vi "Main_TopLevel_1.vi"() -> ()   [LabVIEW 2010]
doc: "Use this template to create an application that executes until you click the Stop button. Unlike the Single Loop Application VI that uses polling, this VI uses the Event Structure."
uses:
  Main_cluster.ctl
  PI E710 Stage.lvlib
panel:
  in  "Center cursor":bool
  in  "Skip scan":bool
  out "Timetrace":dbl[](graph)
  in  "Tab Control":enum32{"Main", "Stage", "Spectrometer"}(tab)
  in  "File":path
  in  "Timetrace length (s)":i32=1024
  in  "Counter Device":tag="APD_Count"
  in  "Acquisition time (s)":dbl=1.0
  in  "Save as":enum16{"", "ASCII", "OriginLab", "Matlab"}(ring)
  in  "Map Geometry":T1
  out "Stage Identification string":string
  out "Position [micrometers]":dbl[](array[numeric]) format="%.6f"
  in  "Scan as cursor":bool
  in  "Position list":dbl[][](array[numeric])
  in  "Stop scan":bool
  in  "Clear list":bool
  in  "Scan":bool
  in  "Move to cursor":bool
  in  "Add to list":bool
  in  "Measure timetraces":bool
  in  "quit":bool
  out "Intensity Graph":dbl[][](graph)
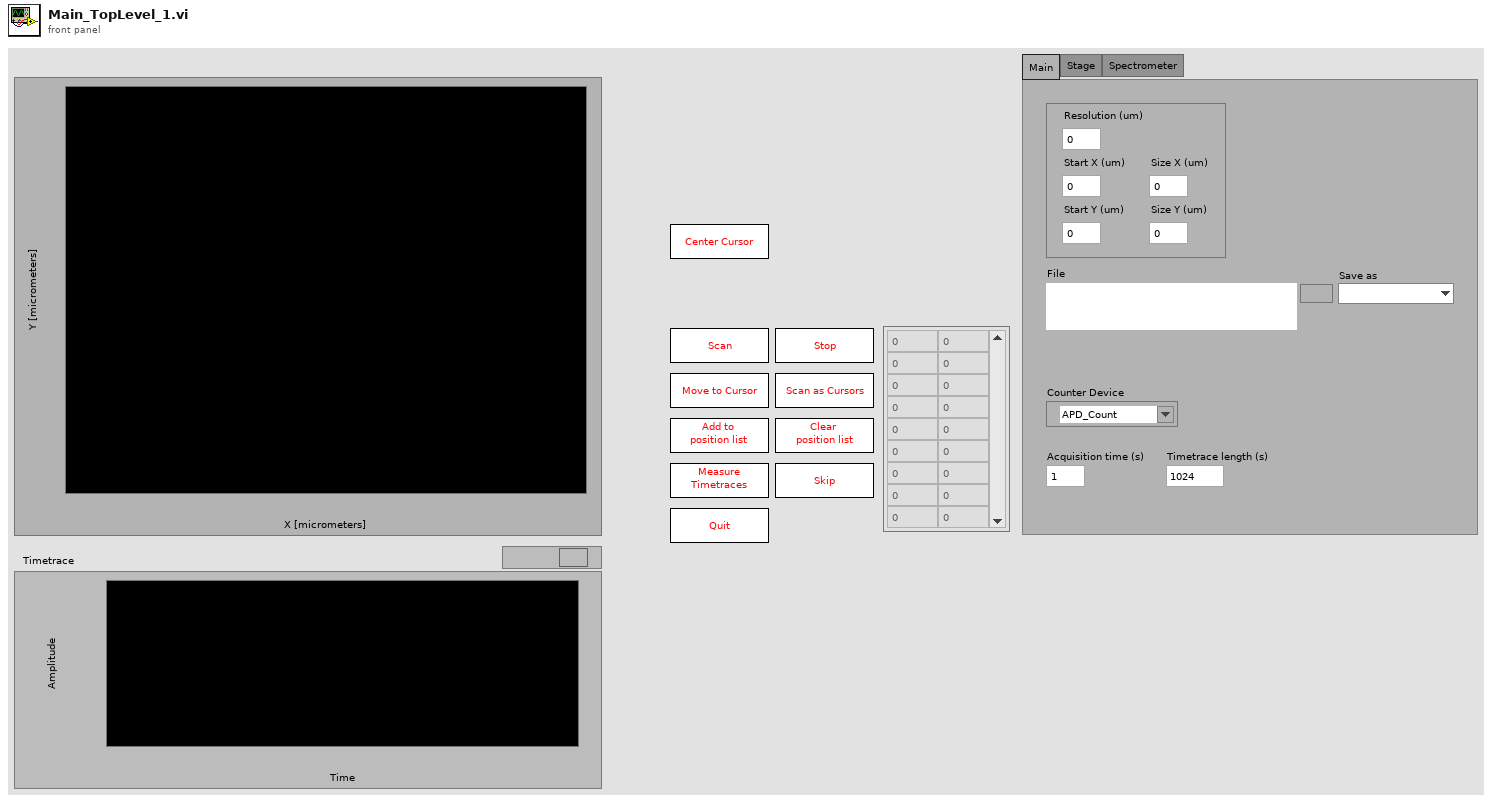
[diagram p1: front panel]
types:
  T1 = cluster{"Size Y (um)":dbl, "Size X (um)":dbl, "Start Y (um)":dbl, "Start X (um)":dbl, "Resolution (um)":dbl}
  T2 = typedef "Main_cluster.ctl" = cluster{"Task array":refnum<k21>[], "Intensity Graph":refnum<vi>, "Timetrace":refnum<vi>, "File output cluster":cluster{"Save as":refnum<vi>, "File":refnum<vi>}, "Skip scan":refnum<vi>, "Stop scan":refnum<vi>, "Acquisition time":dbl}
  T3 = cluster{"Position list[0]":dbl, "Position list[1]":dbl}
  T4 = cluster{"Position list[0]":string, "Position list[1]":string}
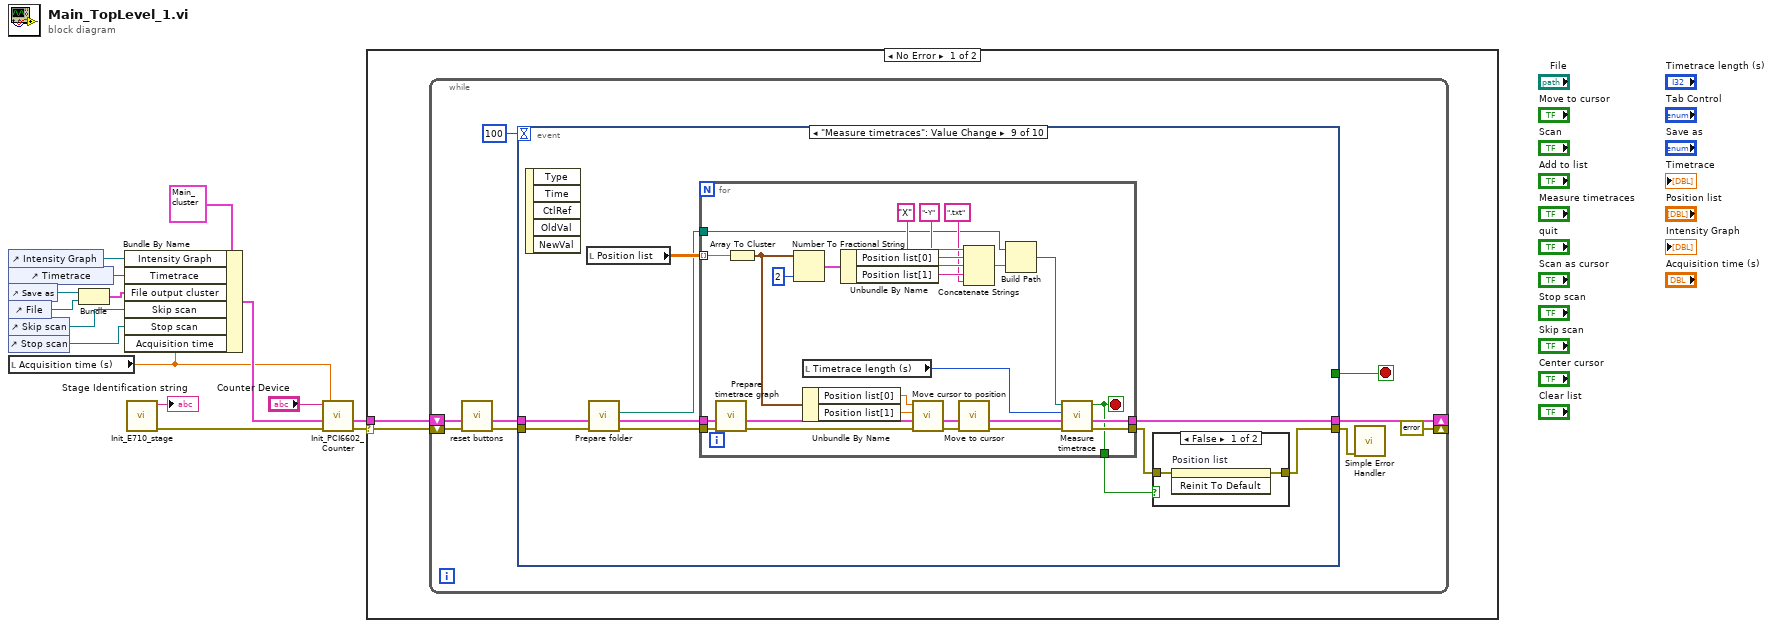
[diagram p0: block diagram]
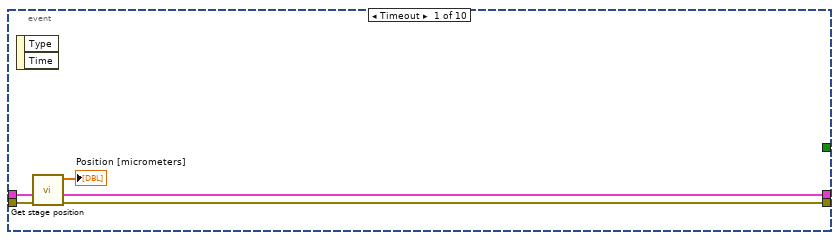
[diagram p2: hidden frame]
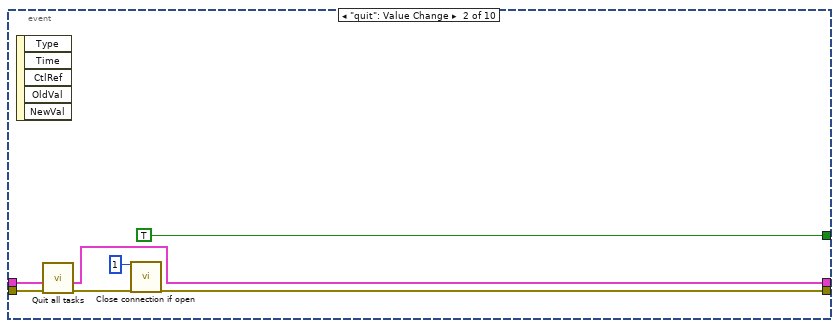
[diagram p3: hidden frame]
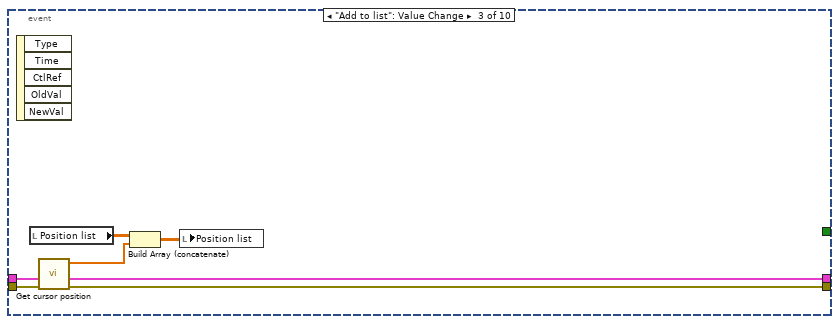
[diagram p4: hidden frame]
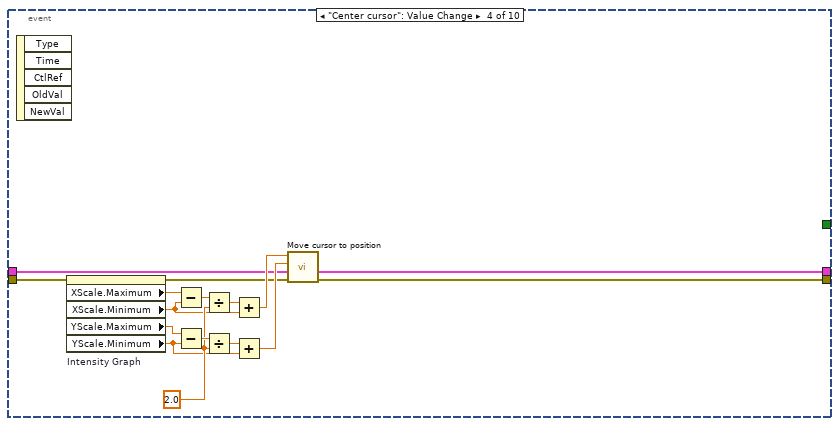
[diagram p5: hidden frame]
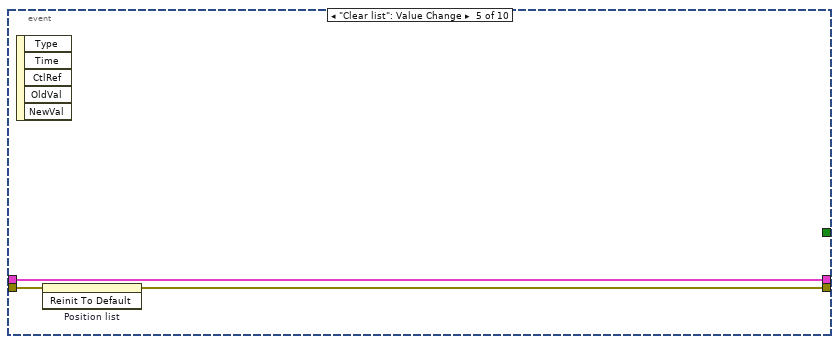
[diagram p6: hidden frame]
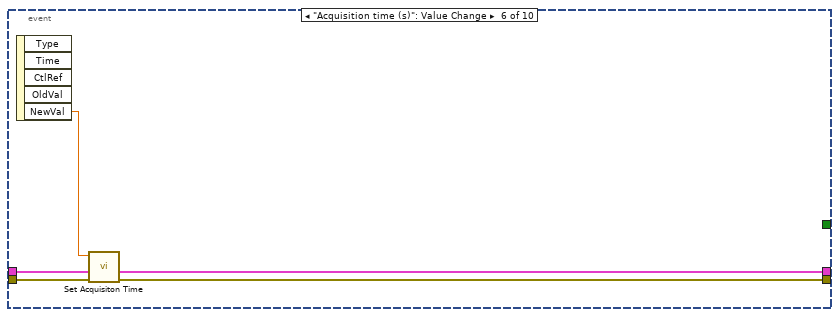
[diagram p7: hidden frame]
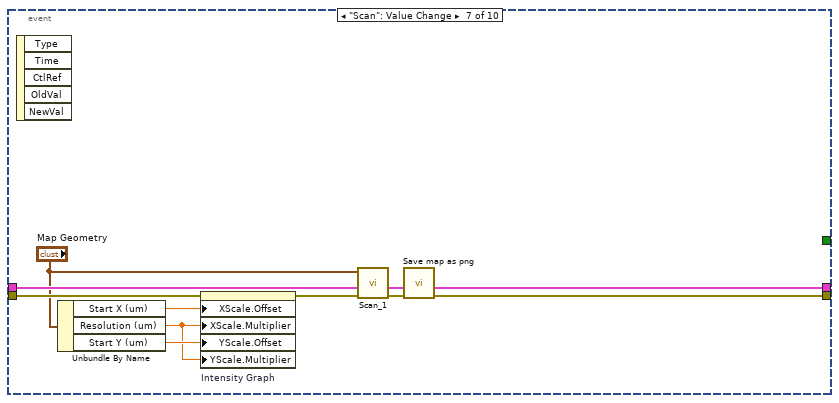
[diagram p8: hidden frame]
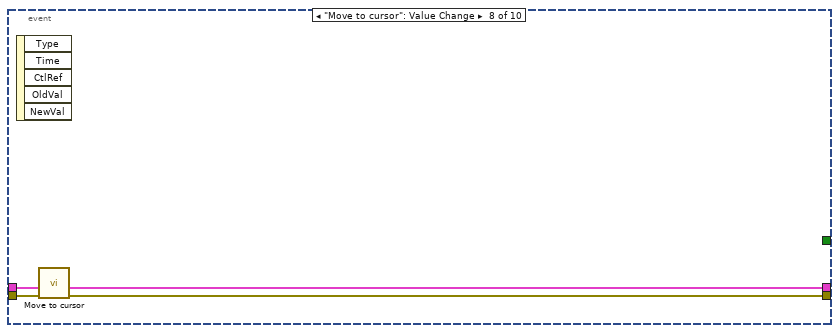
[diagram p9: hidden frame]
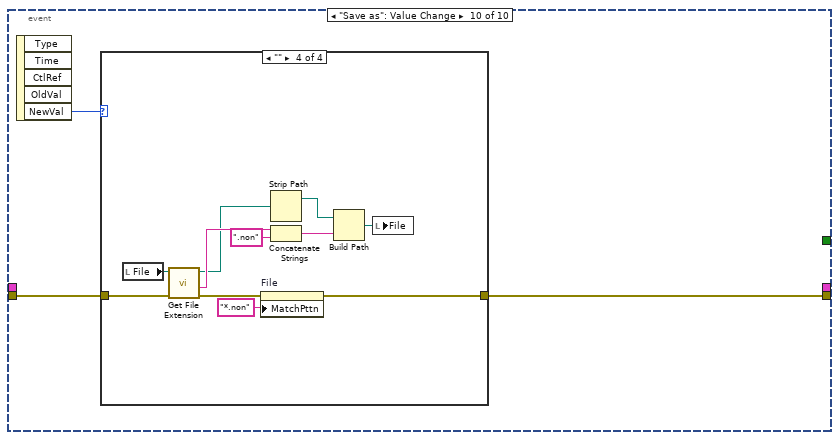
[diagram p11: hidden frame]
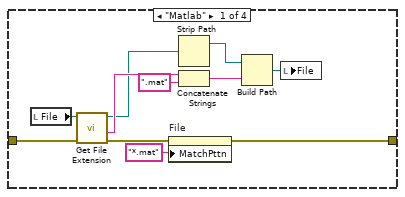
[diagram p12: hidden frame]
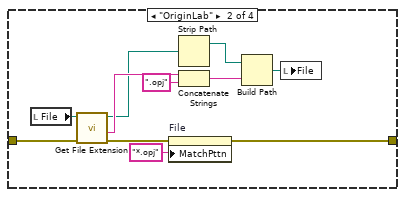
[diagram p13: hidden frame]
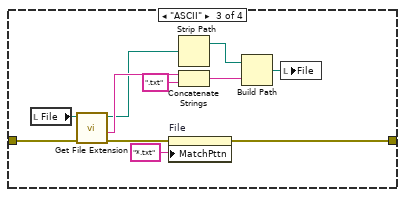
[diagram p14: hidden frame]
diagram:
  n1 = control-ref of="Intensity Graph"() -> (w13:refnum<vi>)
  n2 = control-ref of="Timetrace"() -> (w12:refnum<vi>)
  n3 = control-ref of="Save as"() -> (w11:refnum<vi>)
  n4 = control-ref of="File"() -> (w10:refnum<vi>)
  n5 = control-ref of="Skip scan"() -> (w8:refnum<vi>)
  n6 = control-ref of="Stop scan"() -> (w7:refnum<vi>)
  n7 = local read "Acquisition time (s)"() -> (w1:dbl)
  n8 = Bundle("Save as"=w11, "File"=w10) -> (w9:cluster{"Save as":refnum<vi>, "File":refnum<vi>})  [unwired: 1 in]
  n9 = Bundle By Name(cluster=T2 {"Task array"=[], "Intensity Graph"=refnum, "Timetrace"=refnum, "File output cluster"={"Save as"=refnum, "File"=refnum}, "Skip scan"=refnum, "Stop scan"=refnum, "Acquisition time"=0.0} ("Main cluster"), "Intensity Graph"=w13, "Timetrace"=w12, "File output cluster"=w9, "Skip scan"=w8, "Stop scan"=w7, "Acquisition time"=w1) -> (w3:T2)
  n10 = call "Init_E710_stage.vi"() -> ("error out"=w4:errorcluster, "Stage Identification string"=→"Stage Identification string":string)  [unwired: 6 in]
  n11 = call "Init_PCI6602_Counter.vi"("error in"=w4, "Main cluster"=w3, "Acquisition time (s)"=w1, "Device"="Counter Device") -> ("error out"=w5:errorcluster, "Main cluster"=w2:T2)  [unwired: 2 out]
  n12 = case shown="No Error" w5 {
    selector: w5 -> [w17 _]
    tunnel: w2 -> [w16 _]
    frame No Error {
      n13 = while {
        shift-right: [errorcluster {"status"=FALSE, "code"=0, "source"=""} ("error IO")] -> _
        shift-left: w17 -> [w22]
        shift-right: [w20] -> _
        shift-left: w16 -> [w18]
        stop <- w26 stop-if-true
        n14 = call "reset buttons.vi"("error IO"=w22, "input main cluster"=w18) -> ("error out"=w21:errorcluster, "output main cluster"=w19:T2)  [unwired: 4 in]
        n15 = event shown="[8] \"Measure timetraces\": Value Change" {
          selector: _ -> [_ _ _ _ _ _ _ _ _ _]
          dyn-events: _ -> [_ _ _ _ _ _ _ _ _ _]
          timeout: 100 -> [_ _ _ _ _ _ _ _ _ _]
          tunnel: [_ TRUE ("quit") _ _ _ _ _ _ _ _] -> w26
          tunnel: w21 -> [w30 w36 w40 w48 w63 w68 w74 w83 w88 w123]
          tunnel: [w29 w35 w44 w60 w62 w67 w79 w82 w89 w124] -> w23
          tunnel: w19 -> [w28 w32 w39 w46 w61 w65 w75 w81 w87 _]
          tunnel: [w28 w31 w38 w45 w61 w64 w78 w80 w86 _] -> w20
          event Timeout {
            n16 = event-data() -> ()  [unwired: 1 in, 2 out]
            n17 = call "Get stage position.vi"("error in"=w30) -> ("error out"=w29:errorcluster, "Position [micrometers]"=→"Position [micrometers]":dbl[])  [unwired: 4 in, 1 out]
          }
          event "quit": Value Change {
            n18 = event-data() -> ()  [unwired: 1 in, 5 out]
            n19 = call "Quit all tasks.vi"("error in"=w36, "Main cluster in"=w32) -> ("error out"=w33:errorcluster, "Main cluster out"=w31:T2)  [unwired: 4 in]
            n20 = call "Close connection if open.vi"("System no."=1, "error in"=w33) -> ("error out"=w35:errorcluster)  [unwired: 16 in, 1 out]
          }
          event "Add to list": Value Change {
            n21 = event-data() -> ()  [unwired: 1 in, 5 out]
            n22 = local read "Position list"() -> (w43:dbl[][])
            n23 = call "Get cursor position.vi"("error out"=w40, "input main cluster"=w39) -> ("error out"=w44:errorcluster, "output main cluster"=w38:T2, "Cursor.Cursor Position"=w41:dbl[])  [unwired: 3 in]
            n24 = Build Array (concatenate)(w43, w41) -> (w42:dbl[][])
            n25 = local write "Position list"(w42) -> ()
          }
          event "Center cursor": Value Change {
            w55 = 2.0 ("y")
            n26 = event-data() -> ()  [unwired: 1 in, 5 out]
            n27 = property on="Intensity Graph" class="IntGraph (strict)"(error in=w48) -> (error out=w47:errorcluster, "XScale.Maximum"=w59:dbl, "XScale.Minimum"=w52:dbl, "YScale.Maximum"=w58:dbl, "YScale.Minimum"=w51:dbl)  [unwired: 1 in, 1 out]
            n28 = Subtract(x=w59, y=w52) -> (x-y=w57:dbl)
            n29 = Subtract(x=w58, y=w51) -> (x-y=w56:dbl)
            n30 = Divide(x=w57, y=w55) -> (x/y=w54:dbl)
            n31 = Divide(x=w56, y=w55) -> (x/y=w53:dbl)
            n32 = Add(x=w54, y=w52) -> (x+y=w50:dbl)
            n33 = Add(x=w53, y=w51) -> (x+y=w49:dbl)
            n34 = call "Move cursor to position.vi"("error in"=w47, "input main cluster"=w46, "Y"=w49, "X"=w50) -> ("error out"=w60:errorcluster, "output main cluster"=w45:T2)  [unwired: 2 in]
          }
          event "Clear list": Value Change {
            n35 = event-data() -> ()  [unwired: 1 in, 5 out]
            n36 = invoke on="Position list" class="Arr (strict)" method="Reinit To Default"(error in=w63) -> (error out=w62:errorcluster)  [unwired: 2 in, 2 out]
          }
          event "Acquisition time (s)": Value Change {
            n37 = event-data() -> ("NewVal"=w66:dbl)  [unwired: 1 in, 4 out]
            n38 = call "Set Acquisiton Time.vi"("error in"=w68, "input main cluster"=w65, "Acquisition time"=w66) -> ("error out"=w67:errorcluster, "output main cluster"=w64:T2)  [unwired: 3 in]
          }
          event "Scan": Value Change {
            n39 = event-data() -> ()  [unwired: 1 in, 5 out]
            n40 = Unbundle By Name("Map Geometry") -> ("Start X (um)"=w71:dbl, "Resolution (um)"=w69:dbl, "Start Y (um)"=w70:dbl)
            n41 = property on="Intensity Graph" class="IntGraph (strict)"(error in=w74, "XScale.Offset"=w71, "XScale.Multiplier"=w69, "YScale.Offset"=w70, "YScale.Multiplier"=w69) -> (error out=w73:errorcluster)  [unwired: 1 in, 1 out]
            n42 = call "Scan_1.vi"("error in"=w73, "input main cluster"=w75, "Map geometry"="Map Geometry") -> ("error out"=w77:errorcluster, "output main cluster"=w76:T2)  [unwired: 3 in]
            n43 = call "Save map as png.vi"("error in"=w77, "input main cluster"=w76) -> ("error out"=w79:errorcluster, "output main cluster"=w78:T2)  [unwired: 4 in]
          }
          event "Move to cursor": Value Change {
            n44 = event-data() -> ()  [unwired: 1 in, 5 out]
            n45 = call "Move to cursor.vi"("error in"=w83, "input main cluster"=w81) -> ("error out"=w82:errorcluster, "output main cluster"=w80:T2)  [unwired: 4 in]
          }
          event "Measure timetraces": Value Change {
            n46 = event-data() -> ()  [unwired: 1 in, 5 out]
            n47 = local read "Position list"() -> (w93:dbl[][])
            n48 = call "Prepare folder.vi"("error in"=w88, "input main cluster"=w87) -> ("error out"=w92:errorcluster, "output main cluster"=w85:T2, "created path"=w91:path)  [unwired: 3 in]
            n49 = for {
              tunnel: w93 -> [w112] mode=indexing
              tunnel: w92 -> [w104]
              tunnel: [w111] -> w90
              tunnel: w91 -> [w115]
              tunnel: w85 -> [w101]
              tunnel: [w98] -> w86
              tunnel: [w97] -> w84
              stop <- w97 stop-if-true
              n50 = call "Prepare timetrace graph.vi"("error in"=w104, "input main cluster"=w101) -> ("error out"=w108:errorcluster, "output main cluster"=w99:T2)  [unwired: 4 in]
              n51 = Array To Cluster(array=w112) -> (cluster=w103:T3)
              n52 = Number To Fractional String(number=w103, precision (6)=i16 2) -> (F-format string=w102:T4)  [unwired: 2 in]
              n53 = local read "Timetrace length (s)"() -> (w122:i32)
              n54 = Unbundle By Name(w103) -> ("Position list[0]"=w107:dbl, "Position list[1]"=w106:dbl)
              n55 = Unbundle By Name(w102) -> ("Position list[0]"=w120:string, "Position list[1]"=w118:string)
              n56 = call "Move cursor to position.vi"("error in"=w108, "input main cluster"=w99, "Y"=w106, "X"=w107) -> ("error out"=w109:errorcluster, "output main cluster"=w110:T2)  [unwired: 2 in]
              n57 = call "Move to cursor.vi"("error in"=w109, "input main cluster"=w110) -> ("error out"=w105:errorcluster, "output main cluster"=w100:T2)  [unwired: 4 in]
              n58 = Concatenate Strings("X" ("string"), w120, "-Y" ("string"), w118, ".txt" ("string")) -> (w116:string)
              n59 = Build Path(base path=w115, name or relative path=w116) -> (appended path=w114:path)
              n60 = call "Measure timetrace.vi"("error in"=w105, "input main cluster"=w100, "Timetrace length (s)"=w122, "path"=w114) -> ("error out"=w111:errorcluster, "output main cluster"=w98:T2, "stoped?"=w97:bool)  [unwired: 1 in]
            }
            n61 = case shown="False" w84 {
              tunnel: [w95 w96] -> w89
              tunnel: w90 -> [w94 w96]
              frame False {
                n62 = invoke on="Position list" class="Arr (strict)" method="Reinit To Default"(error in=w94) -> (error out=w95:errorcluster)  [unwired: 2 in, 2 out]
              }
              frame True, Default {
              }
            }
          }
          event "Save as": Value Change {
            n63 = event-data() -> ("NewVal"=w125:enum16{"", "ASCII", "OriginLab", "Matlab"})  [unwired: 1 in, 4 out]
            n64 = case shown="\"\"" w125 {
              tunnel: w123 -> [w133 w144 w155 w166]
              tunnel: [w135 w146 w157 w168] -> w124
              frame "Matlab" {
                n65 = local read "File"() -> (w134:path)
                n66 = call <vilib>:"Get File Extension.vi"("error in (no error)"=w133, "file"=w134) -> ("error out"=w132:errorcluster, "filename without extension"=w131:string, "dup file"=w129:path)  [unwired: 6 in, 1 out]
                n67 = property on="File" class="Path"(error in=w132, "MatchPttn"="*.mat" ("Browse Options:Match Pattern")) -> (error out=w135:errorcluster)  [unwired: 1 in, 1 out]
                n68 = Strip Path(path=w129) -> (stripped path=w128:path)  [unwired: 1 out]
                n69 = Concatenate Strings(w131, ".mat" ("string")) -> (w127:string)
                n70 = Build Path(base path=w128, name or relative path=w127) -> (appended path=w126:path)
                n71 = local write "File"(w126) -> ()
              }
              frame "OriginLab" {
                n72 = local read "File"() -> (w145:path)
                n73 = call <vilib>:"Get File Extension.vi"("error in (no error)"=w144, "file"=w145) -> ("error out"=w143:errorcluster, "filename without extension"=w142:string, "dup file"=w140:path)  [unwired: 6 in, 1 out]
                n74 = property on="File" class="Path"(error in=w143, "MatchPttn"="*.opj" ("Browse Options:Match Pattern")) -> (error out=w146:errorcluster)  [unwired: 1 in, 1 out]
                n75 = Strip Path(path=w140) -> (stripped path=w139:path)  [unwired: 1 out]
                n76 = Concatenate Strings(w142, ".opj" ("string")) -> (w138:string)
                n77 = Build Path(base path=w139, name or relative path=w138) -> (appended path=w137:path)
                n78 = local write "File"(w137) -> ()
              }
              frame "ASCII" {
                n79 = local read "File"() -> (w156:path)
                n80 = call <vilib>:"Get File Extension.vi"("error in (no error)"=w155, "file"=w156) -> ("error out"=w154:errorcluster, "filename without extension"=w153:string, "dup file"=w151:path)  [unwired: 6 in, 1 out]
                n81 = property on="File" class="Path"(error in=w154, "MatchPttn"="*.txt" ("Browse Options:Match Pattern")) -> (error out=w157:errorcluster)  [unwired: 1 in, 1 out]
                n82 = Strip Path(path=w151) -> (stripped path=w150:path)  [unwired: 1 out]
                n83 = Concatenate Strings(w153, ".txt" ("string")) -> (w149:string)
                n84 = Build Path(base path=w150, name or relative path=w149) -> (appended path=w148:path)
                n85 = local write "File"(w148) -> ()
              }
              frame "" {
                n86 = local read "File"() -> (w167:path)
                n87 = call <vilib>:"Get File Extension.vi"("error in (no error)"=w166, "file"=w167) -> ("error out"=w165:errorcluster, "filename without extension"=w164:string, "dup file"=w162:path)  [unwired: 6 in, 1 out]
                n88 = property on="File" class="Path"(error in=w165, "MatchPttn"="*.non" ("Browse Options:Match Pattern")) -> (error out=w168:errorcluster)  [unwired: 1 in, 1 out]
                n89 = Strip Path(path=w162) -> (stripped path=w161:path)  [unwired: 1 out]
                n90 = Concatenate Strings(w164, ".non" ("string")) -> (w160:string)
                n91 = Build Path(base path=w161, name or relative path=w160) -> (appended path=w159:path)
                n92 = local write "File"(w159) -> ()
              }
            }
          }
        }
        n93 = call <vilib>:"Simple Error Handler.vi"("error in (no error)"=w23) -> ()  [unwired: 4 in, 5 out]
      }
    }
    frame Error {
    }
  }
